vi "TDMS Read File.vi"(8 "error in":errorcluster, 9 "Image Index":i64, 10 "Read Settings":T1={"Image Type"=0, "Width"=640, "Height"=480, "Pixels per Image"=337920, "Total Width"=640, "Left Offset"=640, "Image"="test"} {"Image Type" items=["Grayscale (U8)", "Grayscale (I16)", "Grayscale (SGL)", "Complex (CSG)", "RGB (U32)", "HSL (U32)", "RGB (U64)", "Grayscale (U16)"]}, 11 "TDMS Refnum In":refnum<k34>) -> (0 "error out":errorcluster, 1 "read process finished?":bool, 2 "Image":T3, 3 "TDMS Refnum Out":refnum<k34>)   [LabVIEW 2023]
uses:
  <vilib>/vision/Image Controls.llb/IMAQ Image.ctl
  TDMS Read Data.ctl
  TDMS Global.vi
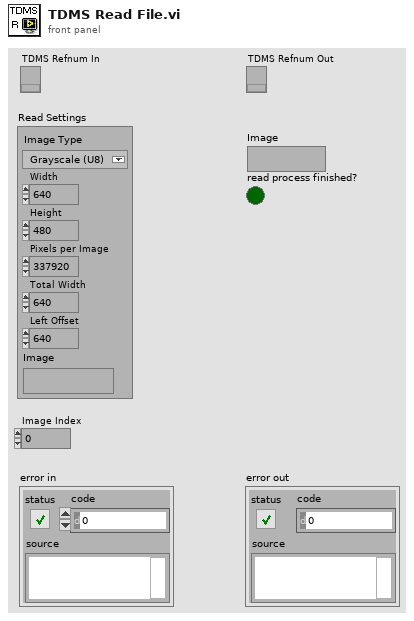
[diagram p1: front panel]
types:
  T1 = typedef "TDMS Read Data.ctl" = cluster{"Image Type":T2, "Width":u32, "Height":u32, "Pixels per Image":u32, "Total Width":u32, "Left Offset":u32, "Image":T3}
  T2 = typedef "Image Type" = u32
  T3 = typedef "IMAQ Image.ctl" = refnum<image>
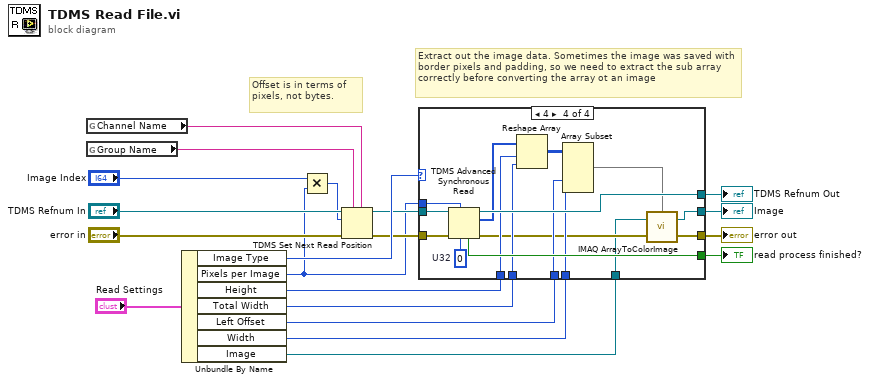
[diagram p0: block diagram]
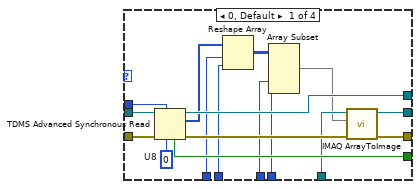
[diagram p2: hidden frame]
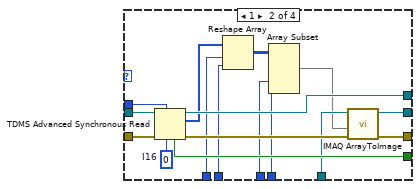
[diagram p3: hidden frame]
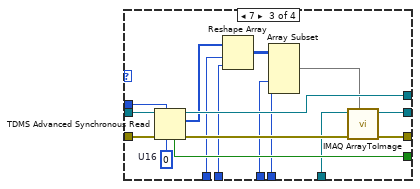
[diagram p4: hidden frame]
diagram:
  # "Extract out the image data. Sometimes the image was saved with border pixels and padding, so we need to extract the sub array correctly before converting the array ot an image"
  # "Offset is in terms of pixels, not bytes."
  n1 = global read "TDMS Global.vi" "Channel Name"() -> (w2:string)
  n2 = global read "TDMS Global.vi" "Group Name"() -> (w1:string)
  n3 = Unbundle By Name("Read Settings") -> ("Image Type"=w17:T2, "Pixels per Image"=w6:u32, "Height"=w8:u32, "Total Width"=w7:u32, "Left Offset"=w5:u32, "Width"=w4:u32, "Image"=w3:T3)
  n4 = Multiply(x="Image Index", y=w6) -> (x*y=w10:i64)
  n5 = TDMS Set Next Read Position(5:w2, 7:w1, 8:"error in", 10:w10, 11:"TDMS Refnum In") -> (0:w13:errorcluster, 3:w12:refnum<k34>)  [unwired: 1 in]
  n6 = case shown="4" w17 {
    tunnel: w12 -> [w36 w53 w70 w87]
    tunnel: w13 -> [w35 w52 w69 w86]
    tunnel: [w33 w50 w67 w84] -> w18
    tunnel: [w28 w45 w62 w75] -> w19
    tunnel: w6 -> [w37 w54 w71 w88]
    tunnel: [w32 w49 w66 w83] -> w16
    tunnel: w8 -> [w29 w46 w63 w81]
    tunnel: w7 -> [w23 w41 w58 w79]
    tunnel: w3 -> [w27 w44 w61 w72]
    tunnel: [w26 w43 w60 w76] -> w20
    tunnel: w5 -> [w22 w40 w57 w78]
    tunnel: w4 -> [w21 w39 w56 w77]
    frame 0, Default {
      w34 = u8 0  # U8
      n7 = TDMS Advanced Synchronous Read(6:w34, 7:w37, 8:w35, 11:w36) -> (0:w30:errorcluster, 2:w31:u8[], 3:w33:refnum<k34>, 4:w32:bool)
      n8 = Reshape Array(w31, w29, w23) -> (w25:u8[][])
      n9 = Array Subset(array=w25, index (col)=w22, length (col)=w21) -> (w24:u8[][])  [unwired: 2 in]
      n10 = call "IMAQ ArrayToImage"("error in (no error)"=w30, "Image Pixels (U8)"=w24, "Image"=w27) -> ("error out"=w28:errorcluster, "Image Out"=w26:T3)  [unwired: 7 in]
    }
    frame 1 {
      w51 = i16 0  # I16
      n11 = TDMS Advanced Synchronous Read(6:w51, 7:w54, 8:w52, 11:w53) -> (0:w47:errorcluster, 2:w48:i16[], 3:w50:refnum<k34>, 4:w49:bool)
      n12 = Reshape Array(w48, w46, w41) -> (w42:i16[][])
      n13 = Array Subset(array=w42, index (col)=w40, length (col)=w39) -> (w38:i16[][])  [unwired: 2 in]
      n14 = call "IMAQ ArrayToImage"("error in (no error)"=w47, "Image Pixels (I16)"=w38, "Image"=w44) -> ("error out"=w45:errorcluster, "Image Out"=w43:T3)  [unwired: 7 in]
    }
    frame 7 {
      w68 = u16 0  # U16
      n15 = TDMS Advanced Synchronous Read(6:w68, 7:w71, 8:w69, 11:w70) -> (0:w64:errorcluster, 2:w65:u16[], 3:w67:refnum<k34>, 4:w66:bool)
      n16 = Reshape Array(w65, w63, w58) -> (w59:u16[][])
      n17 = Array Subset(array=w59, index (col)=w57, length (col)=w56) -> (w55:u16[][])  [unwired: 2 in]
      n18 = call "IMAQ ArrayToImage"("Image Pixels (U16)"=w55, "error in (no error)"=w64, "Image"=w61) -> ("error out"=w62:errorcluster, "Image Out"=w60:T3)  [unwired: 7 in]
    }
    frame 4 {
      w85 = u32 0  # U32
      n19 = TDMS Advanced Synchronous Read(6:w85, 7:w88, 8:w86, 11:w87) -> (0:w74:errorcluster, 2:w82:u32[], 3:w84:refnum<k34>, 4:w83:bool)
      n20 = Reshape Array(w82, w81, w79) -> (w80:u32[][])
      n21 = Array Subset(array=w80, index (col)=w78, length (col)=w77) -> (w73:u32[][])  [unwired: 2 in]
      n22 = call "IMAQ ArrayToColorImage"("Image Pixels (U32)"=w73, "Image"=w72, "error in (no error)"=w74) -> ("Image Out"=w76:T3, "error out"=w75:errorcluster)  [unwired: 2 in]
    }
  }
  "Image" <- w20
  "error out" <- w19
  "TDMS Refnum Out" <- w18
  "read process finished?" <- w16
